vi "GraphPlotCreate.vi"(1 "2D Array input":dbl[][](array[numeric])) -> (0 "Plots output":cluster{dbl[], dbl[]}[](array[cluster]))   [LabVIEW 2021]
panel:
  in  "Meas. Points":i32
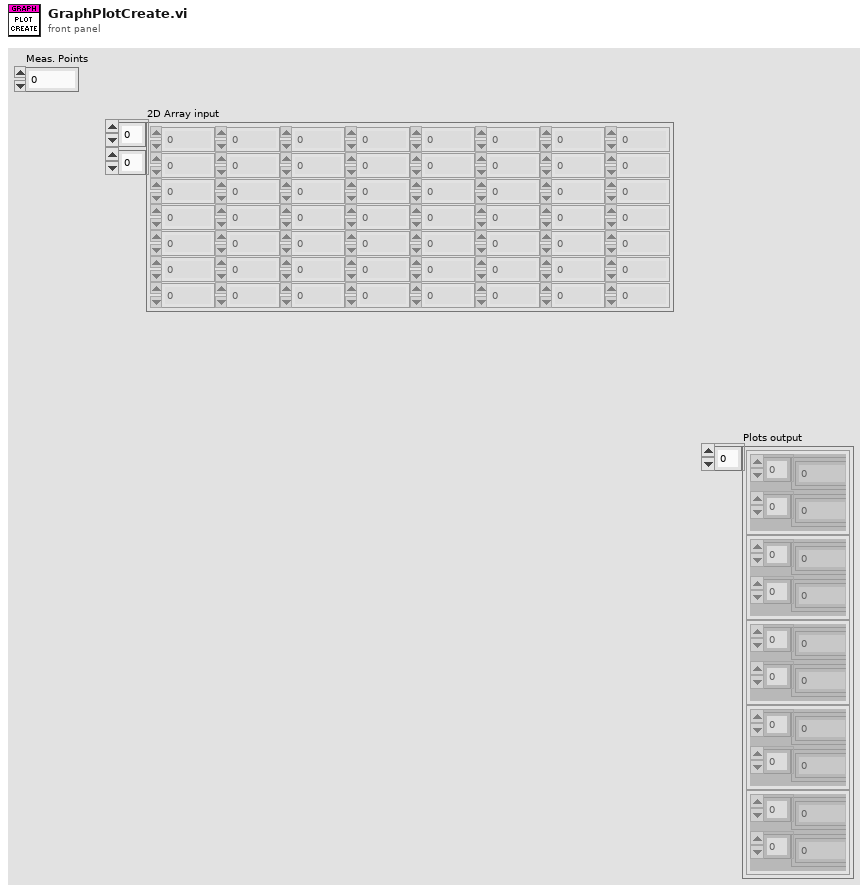
[diagram p1: front panel]
types:
  T1 = cluster{"2D Array input":dbl[], "2D Array input":dbl[]}
  T2 = cluster{"2D Array input":dbl[], "2D Array input":dbl[]}[]
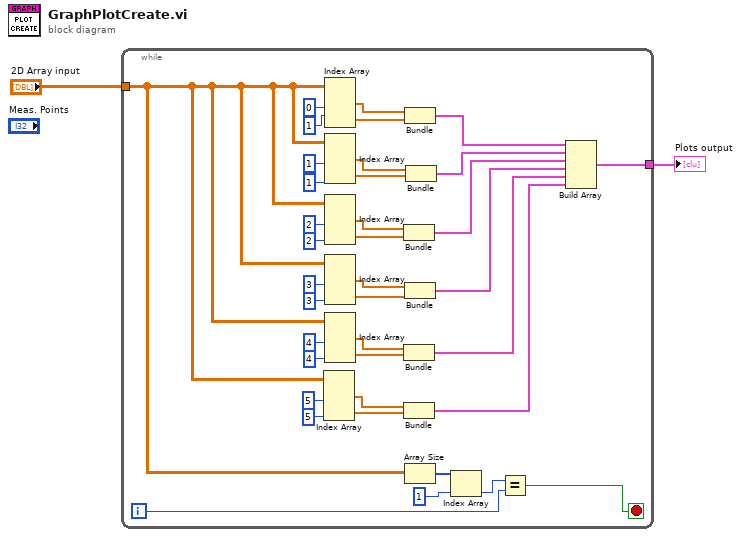
[diagram p0: block diagram]
diagram:
  n1 = while {
    tunnel: [w12] -> w2
    tunnel: "2D Array input" -> [w11]
    i -> [w5]
    stop <- w7 stop-if-true
    n2 = Index Array(array=w11, index (col) #1=5 ("disabled index (col)"), index (col) #2=5 ("index (col)")) -> (element #1=w16:dbl[], element #2=w15:dbl[])  [unwired: 2 in]
    n3 = Index Array(array=w11, index (col) #1=0 ("disabled index (col)"), index (row) #2=1 ("index (col)")) -> (element #1=w36:dbl[], element #2=w35:dbl[])  [unwired: 2 in]
    n4 = Index Array(array=w11, index (col) #1=1 ("index (col)"), index (col) #2=1 ("index (col)")) -> (element #1=w34:dbl[], element #2=w33:dbl[])  [unwired: 2 in]
    n5 = Index Array(array=w11, index (col) #1=2 ("index (col)"), index (col) #2=2 ("index (col)")) -> (element #1=w32:dbl[], element #2=w31:dbl[])  [unwired: 2 in]
    n6 = Index Array(array=w11, index (col) #1=3 ("disabled index (col)"), index (col) #2=3 ("index (col)")) -> (element #1=w20:dbl[], element #2=w19:dbl[])  [unwired: 2 in]
    n7 = Index Array(array=w11, index (col) #1=4 ("disabled index (col)"), index (col) #2=4 ("index (col)")) -> (element #1=w18:dbl[], element #2=w17:dbl[])  [unwired: 2 in]
    n8 = Bundle("2D Array input"=w32, "2D Array input"=w31) -> (w28:T1)  [unwired: 1 in]
    n9 = Bundle("2D Array input"=w18, "2D Array input"=w17) -> (w14:T1)  [unwired: 1 in]
    n10 = Bundle("2D Array input"=w16, "2D Array input"=w15) -> (w13:T1)  [unwired: 1 in]
    n11 = Bundle("2D Array input"=w36, "2D Array input"=w35) -> (w30:T1)  [unwired: 1 in]
    n12 = Bundle("2D Array input"=w20, "2D Array input"=w19) -> (w27:T1)  [unwired: 1 in]
    n13 = Array Size(array=w11) -> (size(s)=w10:i32[])
    n14 = Bundle("2D Array input"=w34, "2D Array input"=w33) -> (w29:T1)  [unwired: 1 in]
    n15 = Index Array(array=w10, index=1) -> (element=w8:i32)
    n16 = Equal?(x=w8, y=w5) -> (x = y?=w7:bool)
    n17 = Build Array(w30, w29, w28, w27, w14, w13) -> (w12:T2)
  }
  "Plots output" <- w2
